vi "KGN Get MFC Gaslist.vi"(8 "Fehler (Eingang, kein Fehler)":errorcluster, 9 "Info Cluster":T1, 10 "VISA-Ressourcenname":refnum<visa-resource-name>, 11 "device (Eingang)":u32) -> (0 "Fehler (Ausgang)":errorcluster, 1 "Info Cluster out":T1, 2 "VISA-Ressourcenname out":refnum<visa-resource-name>, 3 "dup device (Ausgang)":u32, 4 "mfc Gasnamen":string[][](array[string]), 6 "Kommandos gesendet":string)   [LabVIEW 2020, in "Linearisierung v2.lvlib" / "Gasteiler.lvlib" / "HovaCAL_Interface.lvlib" / "KGN.lvlib" / "KGN GUI Get.lvlib"]
uses:
  KGN GUI Get.lvlib
  Controls/Info Cluster.ctl
  get/get.lvlib
  Controls/Controls.lvlib
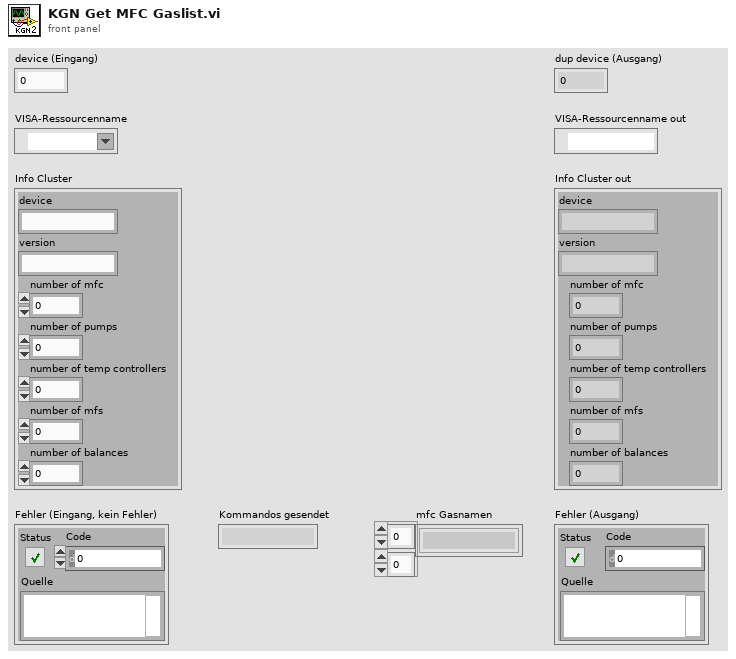
[diagram p1: front panel]
types:
  T1 = typedef "Linearisierung v2.lvlib/Gasteiler.lvlib/HovaCAL_Interface.lvlib/Controls.lvlib/Info Cluster.ctl" = cluster{"device":string, "version":string, "number of mfc":i32, "number of pumps":i32, "number of temp controllers":i32, "number of mfs":i32, "number of balances":i32}
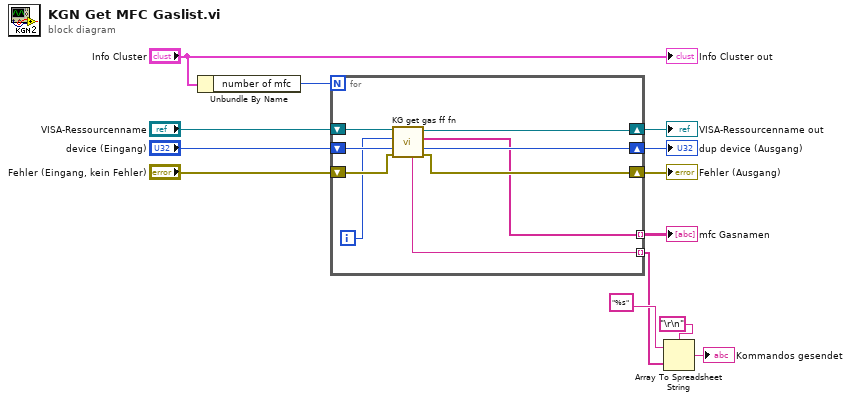
[diagram p0: block diagram]
diagram:
  n1 = Unbundle By Name("Info Cluster") -> ("number of mfc"=w8:i32)
  n2 = for {
    N: w8 -> [_]
    tunnel: [w15] -> w5 mode=indexing
    shift-right: [w16] -> w12
    shift-left: "Fehler (Eingang, kein Fehler)" -> [w21]
    shift-right: [w20] -> w13
    shift-left: "device (Eingang)" -> [w20]
    shift-right: [w18] -> w6
    shift-left: "VISA-Ressourcenname" -> [w19]
    tunnel: [w14] -> w2 mode=indexing
    i -> [w17]
    n3 = call "KG get gas ff fn.vi"("Fehler (Eingang, kein Fehler)"=w21, "mfc"=w17, "VISA-Ressourcenname"=w19) -> ("Fehler (Ausgang)"=w16:errorcluster, "gasnamen"=w15:string[], "VISA-Ressourcenname (Ausgang)"=w18:refnum<visa-resource-name>, "Kommandos gesendet"=w14:string)  [unwired: 5 in]
  }
  "dup device (Ausgang)" <- w13
  "Fehler (Ausgang)" <- w12
  "VISA-Ressourcenname out" <- w6
  "mfc Gasnamen" <- w5
  n4 = Array To Spreadsheet String(delimiter (Tab)="\r\n", array=w2, 3:"%s" ("Format-String")) -> (spreadsheet string=→"Kommandos gesendet":string)
  "Info Cluster out" <- "Info Cluster"
